vi "Calibration.vi"() -> ()   [LabVIEW 2011]
uses:
  <vilib>/Analysis/Matrix/Datatypes/RealMatrix.ctl
  <vilib>/Analysis/_algsub.llb/Real PseudoInverse Matrix.vi
  <vilib>/Analysis/Matrix/Numeric/Multiply/Multiply - RM,RM.vi
  <vilib>/Analysis/baseanly.llb/A x Vector.vi
  <vilib>/Utility/file.llb/Write To Spreadsheet File (DBL).vi
  <vilib>/Analysis/NI_AALBase.lvlib
  <vilib>/Analysis/NI_AALPro.lvlib
  <vilib>/Analysis/Matrix/NI_Matrix.lvlib
panel:
  in  "Radio Buttons":enum32{"Radio Selection 1", "Radio Selection 2"}(radio)
  in  "Z":dbl
  in  "Y":dbl
  in  "X":dbl
  out "Calibrated RGB":string
  out "Reference RGB":string
  out "Calibrated":string
  out "Measured":string
  out "Reference":string
  out "Number of Samples":dbl
  out "XYZ measurements":T1
  out "XYZ references":T1 format="%#.1g"
  in  "Close":bool
  in  "Save":bool
  in  "Test":bool
  in  "Reset":bool
  in  "Capture":bool
  in  "G":u8(slide)=127 scale=0.0..255.0
  in  "B":u8(slide)=127 scale=0.0..255.0
  in  "R":u8(slide)=126 scale=0.0..255.0
  out "Ref Color":u32(colorbox)
  out "Calibration matrix":T1
  out "Meas Color":u32(colorbox)
  in  "XYZ array":dbl[](array[numeric])
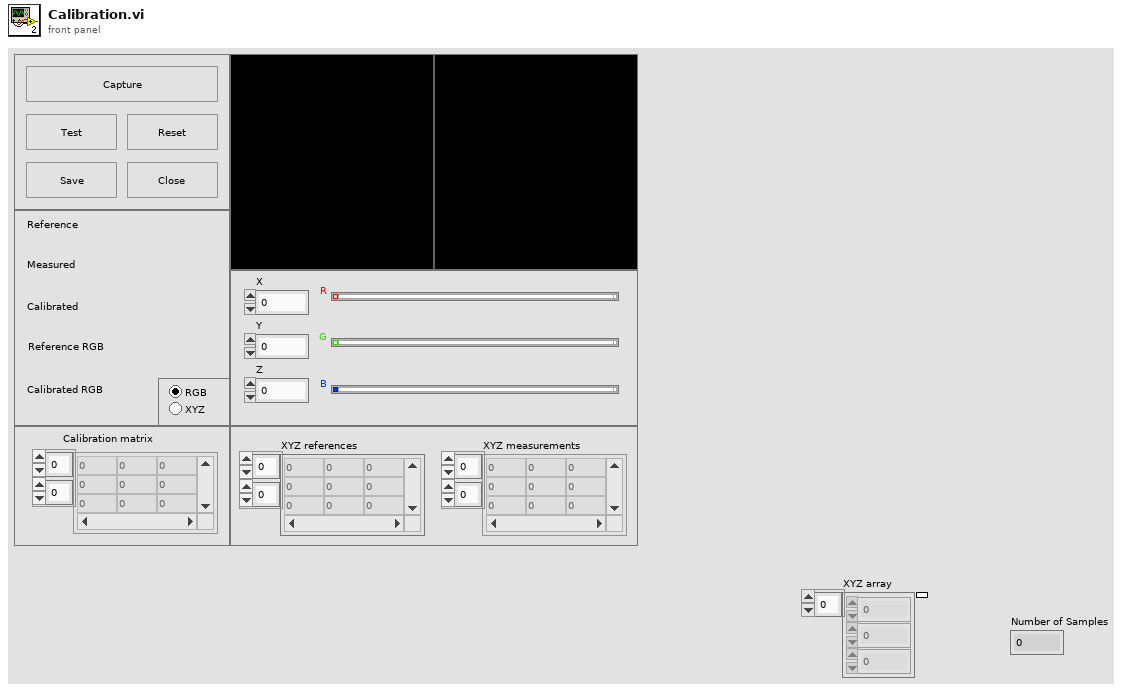
[diagram p1: front panel]
types:
  T1 = typedef "NI_Matrix.lvlib/RealMatrix.ctl" = dbl[][]
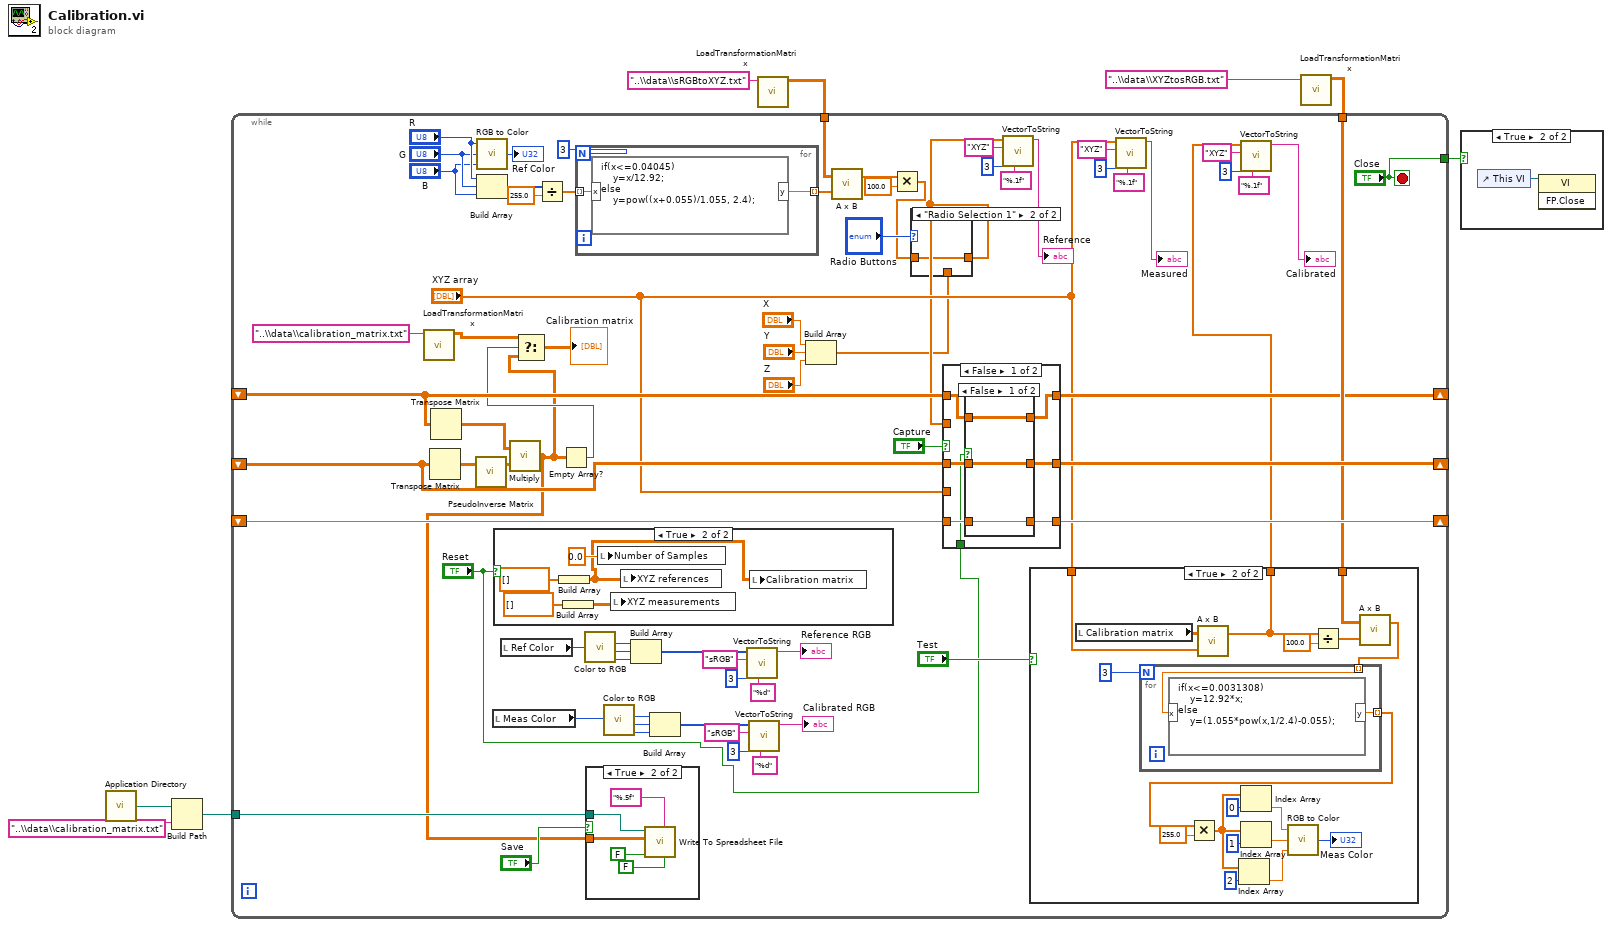
[diagram p0: block diagram]
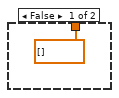
[diagram p5: hidden frame]
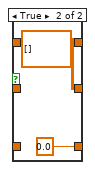
[diagram p7: hidden frame]
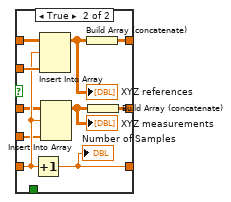
[diagram p8: hidden frame]
diagram:
  n1 = call <vilib>:"Application Directory.vi"() -> ("Application Directory"=w2:path)
  n2 = Build Path(base path=w2, name or relative path="..\\data\\calibration_matrix.txt") -> (appended path=w1:path)
  n3 = call "LoadTransformationMatrix.vi"("relative path"="..\\data\\sRGBtoXYZ.txt" ("name or relative path")) -> ("transformation matrix"=w5:T1)  [unwired: 10 in]
  n4 = call "LoadTransformationMatrix.vi"("relative path"="..\\data\\XYZtosRGB.txt" ("name or relative path")) -> ("transformation matrix"=w6:T1)  [unwired: 10 in]
  n5 = while {
    shift-right: [w78] -> _
    shift-left: _ -> [w67]
    shift-right: [w58] -> _
    shift-left: _ -> [w68]
    shift-right: [w77] -> _
    shift-left: _ -> [w66]
    tunnel: w6 -> [w62]
    tunnel: w5 -> [w60]
    tunnel: ["Close"] -> w4
    tunnel: w1 -> [w23]
    stop <- "Close" stop-if-true
    n6 = call "LoadTransformationMatrix.vi"("relative path"="..\\data\\calibration_matrix.txt" ("name or relative path")) -> ("transformation matrix"=w9:T1)  [unwired: 10 in]
    n7 = Transpose Matrix(1:w66) -> (0:w65:T1)
    n8 = Transpose Matrix(1:w68) -> (0:w63:T1)
    n9 = call-poly <vilib>:"PseudoInverse Matrix.vi"("Input Matrix"=w65) -> ("PseudoInverse Matrix"=w64:T1)  [unwired: 1 in, 1 out]
    n10 = call <vilib>:"RGB to Color.vi"("B"="B", "G"="G", "R"="R") -> ("Color"=→"Ref Color":u32)
    n11 = Build Array("R", "G", "B") -> (w75:u8[])
    n12 = local read "Meas Color"() -> (w24:u32)
    n13 = case shown="True" "Reset" {
      frame False {
      }
      frame True {
        n14 = Build Array(dbl[] [] ("element")) -> (w109:T1)
        n15 = Build Array(dbl[] [] ("element")) -> (w111:T1)
        n16 = local write "Number of Samples"(0.0 ("Numeric")) -> ()
        n17 = local write "XYZ measurements"(w111) -> ()
        n18 = local write "XYZ references"(w109) -> ()
        n19 = local write "Calibration matrix"(w109) -> ()
      }
    }
    n20 = local read "Ref Color"() -> (w41:u32)
    n21 = call-poly <vilib>:"Multiply.vi"("Real Matrix B"=w64, "Real Matrix A"=w63) -> ("A * B"=w12:T1)
    n22 = Divide(x=w75, y=255.0 ("Label Offset.Y")) -> (x/y=w71:dbl[])
    n23 = Empty Array?(array=w12) -> (empty?=w13:bool)
    n24 = Select(t=w9, s=w13, f=w12) -> (s? t:f=→"Calibration matrix":T1)
    n25 = for {
      N: 3 -> [_]
      tunnel: w71 -> [w137] mode=indexing
      tunnel: [w136] -> w61 mode=indexing
      n26 = formula code="if(x<=0.04045)\n    y=x/12.92;\nelse\n    y=pow((x+0.055)/1.055, 2.4);"("x"=w137) -> ("y"=w136:dbl)
    }
    n27 = call <vilib>:"Color to RGB.vi"("Color"=w41) -> ("R"=w40:u8, "G"=w39:u8, "B"=w38:u8)  [unwired: 1 out]
    n28 = case shown="True" "Save" {
      tunnel: w23 -> [_ w84]
      tunnel: w12 -> [_ w83]
      frame False {
      }
      frame True {
        n29 = call-poly <vilib>:"Write To Spreadsheet File.vi"("transpose? (no:F)"=FALSE, "format (%.3f)"="%.5f", "append to file? (new file:F)"=FALSE, "2D data"=w83, "file path (dialog if empty)"=w84) -> ()  [unwired: 3 in, 1 out]
      }
    }
    n30 = call <vilib>:"Color to RGB.vi"("Color"=w24) -> ("R"=w28:u8, "G"=w27:u8, "B"=w26:u8)  [unwired: 1 out]
    n31 = Build Array(w40, w39, w38) -> (w33:u8[])
    n32 = Build Array(w28, w27, w26) -> (w25:u8[])
    n33 = call "VectorToString.vi"("format"="%d", "vector length"=3, "name"="sRGB", "vector"=w33) -> ("string"=→"Reference RGB":string)  [unwired: 7 in]
    n34 = call "VectorToString.vi"("format"="%d", "vector length"=3, "name"="sRGB", "vector"=w25) -> ("string"=→"Calibrated RGB":string)  [unwired: 7 in]
    n35 = Build Array("X", "Y", "Z") -> (w14:dbl[])
    n36 = call-poly <vilib>:"A x B.vi"("Vector"=w61, "A"=w60) -> ("A x Vector"=w69:dbl[])  [unwired: 1 out]
    n37 = Multiply ("Multiply.vi")(x=w69, y=100.0 ("Label Offset.Y")) -> (x*y=w19:dbl[])
    n38 = case shown="\"Radio Selection 1\"" "Radio Buttons" {
      tunnel: w19 -> [_ w82]
      tunnel: [w81 w82] -> w18
      tunnel: w14 -> [w81 _]
      frame "Radio Selection 2", Default {
      }
      frame "Radio Selection 1" {
      }
    }
    n39 = case shown="False" "Capture" {
      tunnel: w18 -> [_ w134]
      tunnel: w68 -> [w115 w135]
      tunnel: [w118 w130] -> w78
      tunnel: w67 -> [w117 w133]
      tunnel: [w120 w128] -> w58
      tunnel: "XYZ array" -> [_ w132]
      tunnel: w66 -> [w116 w131]
      tunnel: [w119 w126] -> w77
      tunnel: "Reset" -> [w114 _]
      frame False {
        n40 = case shown="False" w114 {
          tunnel: [w121 w125] -> w120
          tunnel: [w122 w125] -> w119
          tunnel: [w123 0.0] -> w118
          tunnel: w117 -> [w123 _]
          tunnel: w116 -> [w122 _]
          tunnel: w115 -> [w121 _]
          frame False {
          }
          frame True {
            w125 = T1 [] ("output array")
          }
        }
      }
      frame True {
        n41 = Increment(x=w133) -> (x+1=w130:dbl)
        "Number of Samples" <- w130
        n42 = Insert Into Array(array=w135, index (row)=w133, new element=w134) -> (w129:T1)  [unwired: 1 in]
        "XYZ references" <- w129
        n43 = Insert Into Array(array=w131, index (row)=w133, new element=w132) -> (w127:T1)  [unwired: 1 in]
        "XYZ measurements" <- w127
        n44 = Build Array (concatenate)(w129) -> (w128:T1)
        n45 = Build Array (concatenate)(w127) -> (w126:T1)
      }
    }
    n46 = call "VectorToString.vi"("format"="%.1f", "vector length"=3, "name"="XYZ", "vector"=w18) -> ("string"=→"Reference":string)  [unwired: 7 in]
    n47 = case shown="True" "Test" {
      tunnel: "XYZ array" -> [_ w105]
      tunnel: w62 -> [_ w91]
      tunnel: [dbl[] [] ("A x Vector") w89] -> w45
      frame False {
      }
      frame True {
        n48 = local read "Calibration matrix"() -> (w106:T1)
        n49 = call-poly <vilib>:"A x B.vi"("Vector"=w105, "A"=w106) -> ("A x Vector"=w89:dbl[])  [unwired: 1 out]
        n50 = Divide(x=w89, y=100.0 ("Label Offset.Y")) -> (x/y=w92:dbl[])
        n51 = call-poly <vilib>:"A x B.vi"("Vector"=w92, "A"=w91) -> ("A x Vector"=w90:dbl[])  [unwired: 1 out]
        n52 = for {
          N: 3 -> [_]
          tunnel: w90 -> [w108] mode=indexing
          tunnel: [w107] -> w93 mode=indexing
          n53 = formula code="if(x<=0.0031308)\n    y=12.92*x;\nelse\n    y=(1.055*pow(x,1/2.4)-0.055);"("x"=w108) -> ("y"=w107:dbl)
        }
        n54 = Multiply ("Multiply.vi")(x=w93, y=255.0 ("Label Offset.Y")) -> (x*y=w96:dbl[])
        n55 = Index Array(array=w96, index=2) -> (element=w97:dbl)
        n56 = Index Array(array=w96, index=0) -> (element=w98:dbl)
        n57 = Index Array(array=w96, index=1) -> (element=w95:dbl)
        n58 = call <vilib>:"RGB to Color.vi"("B"=w97, "G"=w95, "R"=w98) -> ("Color"=→"Meas Color":u32)
      }
    }
    n59 = call "VectorToString.vi"("format"="%.1f", "vector length"=3, "name"="XYZ", "vector"="XYZ array") -> ("string"=→"Measured":string)  [unwired: 7 in]
    n60 = call "VectorToString.vi"("format"="%.1f", "vector length"=3, "name"="XYZ", "vector"=w45) -> ("string"=→"Calibrated":string)  [unwired: 7 in]
  }
  n61 = case shown="True" w4 {
    frame False {
    }
    frame True {
      n62 = control-ref of="This VI"() -> (w138:refnum<vi>)
      n63 = invoke class="VI" method="FP.Close"(reference=w138) -> ()  [unwired: 2 in, 3 out]
    }
  }
